vi "NT Connection Info.vi"() -> (3 "Connected":bool)   [LabVIEW 2025]
doc: "Return basic information about Network Table Connections."
uses:
  ntcoreffi.dll
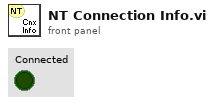
[diagram p1: front panel]
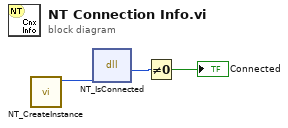
[diagram p0: block diagram]
diagram:
  n1 = call <vilib>:"NT_CreateInstance.vi"() -> ("InstanceHandle"=w1:u64)  [unwired: 10 in, 1 out]
  n2 = dll-call lib="ntcoreffi.*" fn="NT_IsConnected"("InstHandle"=w1) -> ("isConnected"=w3:u32)  [unwired: 4 in, 2 out]
  n3 = Not Equal To 0?(x=w3) -> (x != 0?=→"Connected":bool)
